vi "Find Min Max Position.vi"(4 "Lines with Edges (last)":u32[](array[numeric]), 6 "Lines with Edges (first)":u32[](array[numeric]), 8 "Min / Max":bool, 9 "Search Lines":T1(array[cluster])=[{{"X"=55.0, "Y"=48.0}, {"X"=263.0, "Y"=104.0}}, {{"X"=53.0, "Y"=53.0}, {"X"=262.0, "Y"=109.0}}, {{"X"=52.0, "Y"=58.0}, {"X"=261.0, "Y"=113.0}}, {{"X"=51.0, "Y"=62.0}, {"X"=259.0, "Y"=118.0}}, {{"X"=49.0, "Y"=67.0}, {"X"=258.0, "Y"=123.0}}, {{"X"=48.0, "Y"=72.0}, {"X"=257.0, "Y"=128.0}}, {{"X"=47.0, "Y"=77.0}, {"X"=255.0, "Y"=133.0}}, {{"X"=46.0, "Y"=82.0}, {"X"=254.0, "Y"=138.0}}, {{"X"=44.0, "Y"=87.0}, {"X"=253.0, "Y"=142.0}}, {{"X"=43.0, "Y"=91.0}, {"X"=252.0, "Y"=147.0}}, {{"X"=42.0, "Y"=96.0}, {"X"=250.0, "Y"=152.0}}] {"?"."Y" format="%.2f"; "?"."X" format="%.2f"; "?"."Y" format="%.2f"; "?"."X" format="%.2f"}, 10 "Last Edges":cluster{"X":sgl, "Y":sgl}[](array[cluster])=[{"X"=67.0, "Y"=51.0}, {"X"=230.0, "Y"=95.0}, {"X"=66.0, "Y"=56.0}, {"X"=230.0, "Y"=100.0}, {"X"=66.0, "Y"=62.0}, {"X"=230.0, "Y"=105.0}, {"X"=66.0, "Y"=66.0}, {"X"=230.0, "Y"=110.0}, {"X"=65.0, "Y"=71.0}, {"X"=230.0, "Y"=115.0}, {"X"=65.0, "Y"=77.0}, {"X"=230.0, "Y"=121.0}, {"X"=65.0, "Y"=82.0}, {"X"=229.0, "Y"=126.0}, {"X"=65.0, "Y"=87.0}, {"X"=229.0, "Y"=131.0}, {"X"=64.0, "Y"=92.0}, {"X"=229.0, "Y"=136.0}, {"X"=64.0, "Y"=97.0}, {"X"=229.0, "Y"=141.0}, {"X"=64.0, "Y"=102.0}, {"X"=229.0, "Y"=146.0}] {"Y" format="%.2f"; "X" format="%.2f"}, 11 "First Edges":cluster{"X":sgl, "Y":sgl}[](array[cluster])=[{"X"=67.0, "Y"=51.0}, {"X"=230.0, "Y"=95.0}, {"X"=66.0, "Y"=56.0}, {"X"=230.0, "Y"=100.0}, {"X"=66.0, "Y"=62.0}, {"X"=230.0, "Y"=105.0}, {"X"=66.0, "Y"=66.0}, {"X"=230.0, "Y"=110.0}, {"X"=65.0, "Y"=71.0}, {"X"=230.0, "Y"=115.0}, {"X"=65.0, "Y"=77.0}, {"X"=230.0, "Y"=121.0}, {"X"=65.0, "Y"=82.0}, {"X"=229.0, "Y"=126.0}, {"X"=65.0, "Y"=87.0}, {"X"=229.0, "Y"=131.0}, {"X"=64.0, "Y"=92.0}, {"X"=229.0, "Y"=136.0}, {"X"=64.0, "Y"=97.0}, {"X"=229.0, "Y"=141.0}, {"X"=64.0, "Y"=102.0}, {"X"=229.0, "Y"=146.0}] {"Y" format="%.2f"; "X" format="%.2f"}) -> (1 "Distance":sgl format="%.2f", 2 "Perpendicular Lines":T1(array[cluster])=[{{"X"=55.0, "Y"=48.0}, {"X"=263.0, "Y"=104.0}}, {{"X"=53.0, "Y"=53.0}, {"X"=262.0, "Y"=109.0}}, {{"X"=52.0, "Y"=58.0}, {"X"=261.0, "Y"=113.0}}, {{"X"=51.0, "Y"=62.0}, {"X"=259.0, "Y"=118.0}}, {{"X"=49.0, "Y"=67.0}, {"X"=258.0, "Y"=123.0}}, {{"X"=48.0, "Y"=72.0}, {"X"=257.0, "Y"=128.0}}, {{"X"=47.0, "Y"=77.0}, {"X"=255.0, "Y"=133.0}}, {{"X"=46.0, "Y"=82.0}, {"X"=254.0, "Y"=138.0}}, {{"X"=44.0, "Y"=87.0}, {"X"=253.0, "Y"=142.0}}, {{"X"=43.0, "Y"=91.0}, {"X"=252.0, "Y"=147.0}}, {{"X"=42.0, "Y"=96.0}, {"X"=250.0, "Y"=152.0}}] {"?"."Y" format="%.2f"; "?"."X" format="%.2f"; "?"."Y" format="%.2f"; "?"."X" format="%.2f"}, 3 "Points":cluster{"X":sgl, "Y":sgl}[](array[cluster])=[{"X"=67.0, "Y"=51.0}, {"X"=230.0, "Y"=95.0}, {"X"=66.0, "Y"=56.0}, {"X"=230.0, "Y"=100.0}, {"X"=66.0, "Y"=62.0}, {"X"=230.0, "Y"=105.0}, {"X"=66.0, "Y"=66.0}, {"X"=230.0, "Y"=110.0}, {"X"=65.0, "Y"=71.0}, {"X"=230.0, "Y"=115.0}, {"X"=65.0, "Y"=77.0}, {"X"=230.0, "Y"=121.0}, {"X"=65.0, "Y"=82.0}, {"X"=229.0, "Y"=126.0}, {"X"=65.0, "Y"=87.0}, {"X"=229.0, "Y"=131.0}, {"X"=64.0, "Y"=92.0}, {"X"=229.0, "Y"=136.0}, {"X"=64.0, "Y"=97.0}, {"X"=229.0, "Y"=141.0}, {"X"=64.0, "Y"=102.0}, {"X"=229.0, "Y"=146.0}] {"Y" format="%.2f"; "X" format="%.2f"})   [LabVIEW 2020]
uses:
  NI_Vision_Development_Module.lvlib
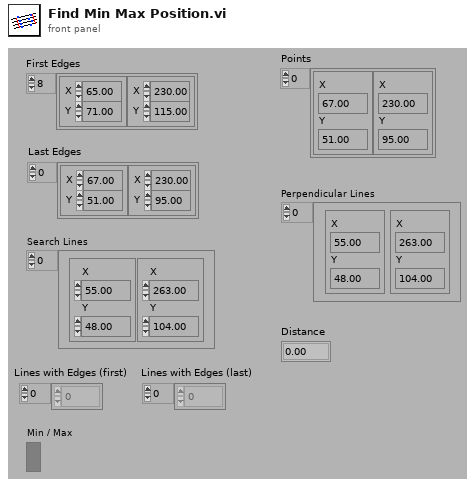
[diagram p1: front panel]
types:
  T1 = cluster{cluster{"X":sgl, "Y":sgl}, cluster{"X":sgl, "Y":sgl}}[]
  T2 = cluster{"(A,B)":cluster{"X":sgl, "Y":sgl}, "(A,B)":cluster{"X":sgl, "Y":sgl}}[]
  T3 = cluster{cluster{"X":sgl, "Y":sgl}, cluster{"X":sgl, "Y":sgl}}
  T4 = cluster{"Point 1":cluster{"X":sgl, "Y":sgl}, "Point 2":cluster{"X":sgl, "Y":sgl}}
  T5 = cluster{"[0]":cluster{"X":sgl, "Y":sgl}, "[1]":cluster{"X":sgl, "Y":sgl}}
  T6 = cluster{"[0]":cluster{"X":sgl, "Y":sgl}, "[1]":cluster{"X":sgl, "Y":sgl}}[]
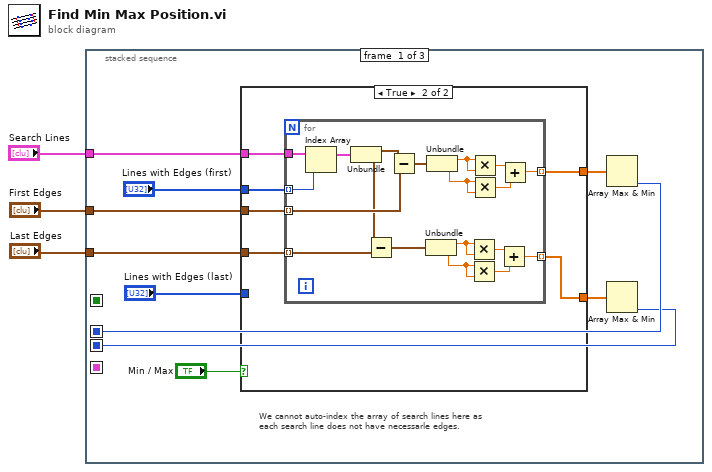
[diagram p0: block diagram]
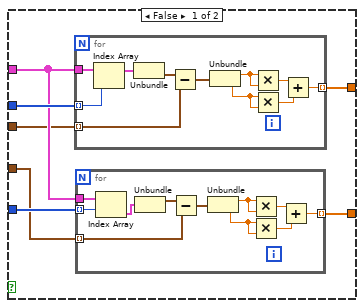
[diagram p2: hidden frame]
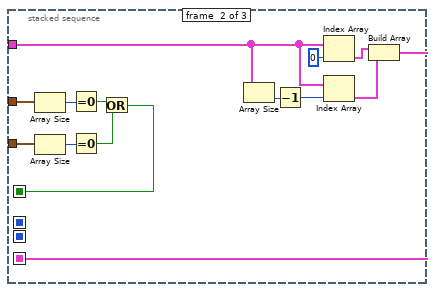
[diagram p3: hidden frame]
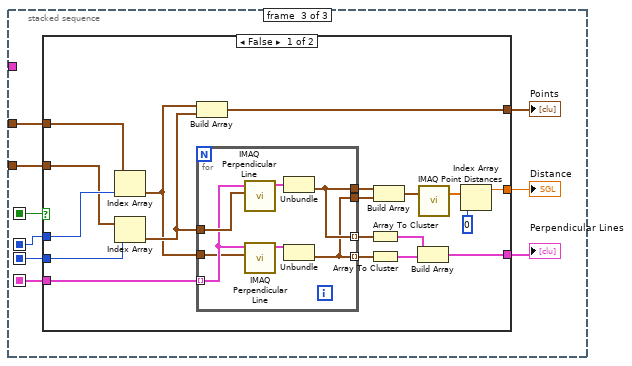
[diagram p4: hidden frame]
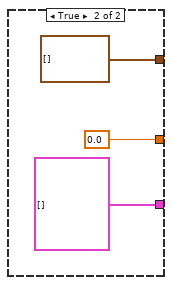
[diagram p5: hidden frame]
diagram:
  n1 = stacked-sequence {
    seq-local: [_ w75 _] -> [_ _ w86]
    seq-local: [w8 _ _] -> [_ _ w85]
    seq-local: [w7 _ _] -> [_ _ w84]
    seq-local: [_ w68 _] -> [_ _ w82]
    tunnel: "Search Lines" -> [w11 w76 _]
    tunnel: "First Edges" -> [w10 w71 w87]
    tunnel: "Last Edges" -> [w9 w74 w83]
    frame #0 {
      # "We cannot auto-index the array of search lines here as\neach search line does not have necessarle edges."
      n2 = case shown="True" "Min / Max" {
        tunnel: [w15 w48] -> w13
        tunnel: [w14 w47] -> w12
        tunnel: w11 -> [w18 w46]
        tunnel: w10 -> [w17 w45]
        tunnel: w9 -> [w16 w44]
        tunnel: "Lines with Edges (first)" -> [w20 w43]
        tunnel: "Lines with Edges (last)" -> [w19 _]
        frame False {
          n3 = for {
            tunnel: w18 -> [w42]
            tunnel: w20 -> [w41] mode=indexing
            tunnel: w17 -> [w39] mode=indexing
            tunnel: [w32] -> w15 mode=indexing
            n4 = Index Array(array=w42, index=w41) -> (element=w40:T3)
            n5 = Unbundle(w40) -> (w38:cluster{"X":sgl, "Y":sgl})  [unwired: 1 out]
            n6 = Subtract(x=w38, y=w39) -> (x-y=w33:cluster{"X":sgl, "Y":sgl})
            n7 = Unbundle(w33) -> ("X"=w34:sgl, "Y"=w35:sgl)
            n8 = Multiply(x=w34, y=w34) -> (x*y=w36:sgl)
            n9 = Multiply(x=w35, y=w35) -> (x*y=w37:sgl)
            n10 = Add(x=w36, y=w37) -> (x+y=w32:sgl)
          }
          n11 = for {
            tunnel: w19 -> [w28] mode=indexing
            tunnel: w18 -> [w29]
            tunnel: w16 -> [w27] mode=indexing
            tunnel: [w21] -> w14 mode=indexing
            n12 = Index Array(array=w29, index=w28) -> (element=w31:T3)
            n13 = Unbundle(w31) -> (w30:cluster{"X":sgl, "Y":sgl})  [unwired: 1 out]
            n14 = Subtract(x=w30, y=w27) -> (x-y=w22:cluster{"X":sgl, "Y":sgl})
            n15 = Unbundle(w22) -> ("X"=w23:sgl, "Y"=w24:sgl)
            n16 = Multiply(x=w23, y=w23) -> (x*y=w25:sgl)
            n17 = Multiply(x=w24, y=w24) -> (x*y=w26:sgl)
            n18 = Add(x=w25, y=w26) -> (x+y=w21:sgl)
          }
        }
        frame True {
          n19 = for {
            tunnel: w45 -> [w67] mode=indexing
            tunnel: w44 -> [w66] mode=indexing
            tunnel: w46 -> [w65]
            tunnel: [w55] -> w48 mode=indexing
            tunnel: [w49] -> w47 mode=indexing
            tunnel: w43 -> [w64] mode=indexing
            n20 = Index Array(array=w65, index=w64) -> (element=w63:T3)
            n21 = Unbundle(w63) -> (w62:cluster{"X":sgl, "Y":sgl}, w61:cluster{"X":sgl, "Y":sgl})
            n22 = Subtract(x=w61, y=w66) -> (x-y=w50:cluster{"X":sgl, "Y":sgl})
            n23 = Subtract(x=w62, y=w67) -> (x-y=w60:cluster{"X":sgl, "Y":sgl})
            n24 = Unbundle(w50) -> ("X"=w51:sgl, "Y"=w52:sgl)
            n25 = Unbundle(w60) -> ("X"=w59:sgl, "Y"=w58:sgl)
            n26 = Multiply(x=w51, y=w51) -> (x*y=w53:sgl)
            n27 = Multiply(x=w52, y=w52) -> (x*y=w54:sgl)
            n28 = Multiply(x=w59, y=w59) -> (x*y=w57:sgl)
            n29 = Multiply(x=w58, y=w58) -> (x*y=w56:sgl)
            n30 = Add(x=w53, y=w54) -> (x+y=w49:sgl)
            n31 = Add(x=w57, y=w56) -> (x+y=w55:sgl)
          }
        }
      }
      n32 = Array Max & Min(array=w13) -> (min index (indices)=w8:i32)  [unwired: 3 out]
      n33 = Array Max & Min(array=w12) -> (min index (indices)=w7:i32)  [unwired: 3 out]
    }
    frame #1 {
      n34 = Array Size(array=w71) -> (size(s)=w72:i32)
      n35 = Array Size(array=w74) -> (size(s)=w73:i32)
      n36 = Equal To 0?(x=w72) -> (x = 0?=w70:bool)
      n37 = Equal To 0?(x=w73) -> (x = 0?=w69:bool)
      n38 = Or(x=w70, y=w69) -> (x .or. y?=w68:bool)
      n39 = Array Size(array=w76) -> (size(s)=w81:i32)
      n40 = Decrement(x=w81) -> (x-1=w80:i32)
      n41 = Index Array(array=w76, index=0 ("Index")) -> (element=w79:T3)
      n42 = Index Array(array=w76, index=w80) -> (element=w78:T3)
      n43 = Build Array(w79, w78) -> (w75:T1)
    }
    frame #2 {
      n44 = case shown="False" w82 {
        tunnel: [w108 T2 []] -> w90
        tunnel: [w92 0.0] -> w89
        tunnel: [w103 cluster{"X":sgl, "Y":sgl}[] []] -> w88
        tunnel: w87 -> [w102 _]
        tunnel: w86 -> [w101 _]
        tunnel: w85 -> [w100 _]
        tunnel: w84 -> [w99 _]
        tunnel: w83 -> [w98 _]
        frame False {
          n45 = Index Array(array=w102, index=w100) -> (element=w97:cluster{"X":sgl, "Y":sgl})
          n46 = Index Array(array=w98, index=w99) -> (element=w109:cluster{"X":sgl, "Y":sgl})
          n47 = Build Array(w97, w109) -> (w103:cluster{"X":sgl, "Y":sgl}[])
          n48 = for {
            tunnel: w101 -> [w113] mode=indexing
            tunnel: w109 -> [w114]
            tunnel: [w115] -> w104 mode=indexing
            tunnel: [w111] -> w105 mode=indexing
            tunnel: [w115] -> w96
            tunnel: [w111] -> w95
            tunnel: w97 -> [w110]
            n49 = call "IMAQ Perpendicular Line"("Point"=w114, "Line"=w113) -> ("Perpendicular Line"=w116:T4)  [unwired: 7 in, 2 out]
            n50 = call "IMAQ Perpendicular Line"("Point"=w110, "Line"=w113) -> ("Perpendicular Line"=w112:T4)  [unwired: 7 in, 2 out]
            n51 = Unbundle(w116) -> ("Point 2"=w115:cluster{"X":sgl, "Y":sgl})  [unwired: 1 out]
            n52 = Unbundle(w112) -> ("Point 2"=w111:cluster{"X":sgl, "Y":sgl})  [unwired: 1 out]
          }
          n53 = Array To Cluster(array=w104) -> (cluster=w106:T5)
          n54 = Array To Cluster(array=w105) -> (cluster=w107:T5)
          n55 = Build Array(w96, w95) -> (w94:cluster{"X":sgl, "Y":sgl}[])
          n56 = Build Array(w106, w107) -> (w108:T6)
          n57 = call "IMAQ Point Distances"("Points"=w94) -> ("Distances"=w93:sgl[])  [unwired: 4 in, 1 out]
          n58 = Index Array(array=w93, index=0 ("Index")) -> (element=w92:sgl)
        }
        frame True {
        }
      }
      "Distance" <- w89
      "Perpendicular Lines" <- w90
      "Points" <- w88
    }
  }
